vi "CleanupCallback.vi"(8 "error in (no error)":errorcluster, 11 "References":T1) -> (0 "error out":errorcluster)   [LabVIEW 2011]
uses:
  FunctionPointerProxy/LabVIEW/t_CallbackReferences.ctl
  C:/Users/Behavior Room/Desktop/Kinect Mouse/DepthSense/FunctionPointerProxy/FunctionPointerProxy/bin/Release/FunctionPointerProxy.dll
  FunctionPointerProxy/FunctionPointerProxy/bin/Release/FunctionPointerProxy.dll
panel:
  # "//Copyright (c) 2006 Bruno van Dooren\n//Permission is hereby granted, free of charge, to any person obtaining a copy\n//of this software and associated documentation files (the \"Software\"), to deal\n//in the Software without restriction, including without limitation the rights\n//to use, copy, modify, merge, publish, distribute, sublicense, and/or sell\n//copies of the Software, and to permit persons to whom the Software is\n//furnished to do so, subject to the following conditions:\n//The above copyright notice and this permission notice shall be included in all\n//copies or substantial portions of the Software.\n//THE SOFTWARE IS PROVIDED \"AS IS\", WITHOUT WARRANTY OF ANY KIND, EXPRESS OR\n//IMPLIED, INCLUDING BUT NOT LIMITED TO THE WARRANTIES OF MERCHANTABILITY,\n//FITNESS FOR A PARTICULAR PURPOSE AND NONINFRINGEMENT. IN NO EVENT SHALL THE\n//AUTHORS OR COPYRIGHT HOLDERS BE LIABLE FOR ANY CLAIM, DAMAGES OR OTHER\n//LIABILITY, WHETHER IN AN ACTION OF CONTRACT, TORT OR OTHERWISE, ARISING FROM,\n//OUT OF OR IN CONNECTION WITH THE SOFTWARE OR THE USE OR OTHER DEALINGS IN THE\n//SOFTWARE."
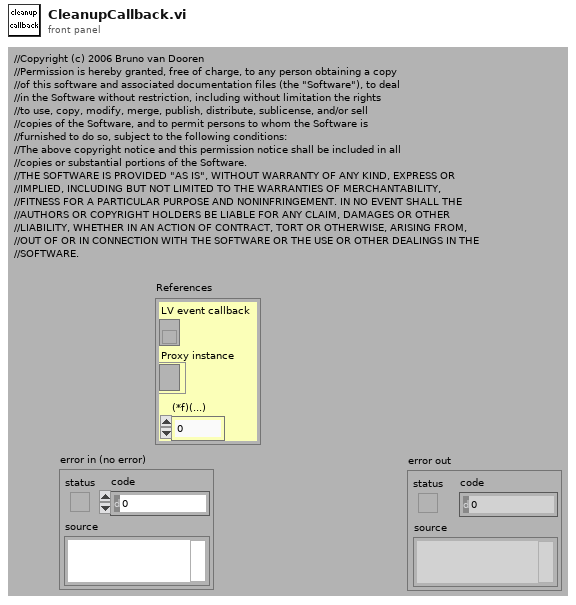
[diagram p1: front panel]
types:
  T1 = typedef "t_CallbackReferences.ctl" = cluster{"LV event callback ":refnum<k27>, "Proxy instance":refnum<k24>, "(*f)(...)":i32}
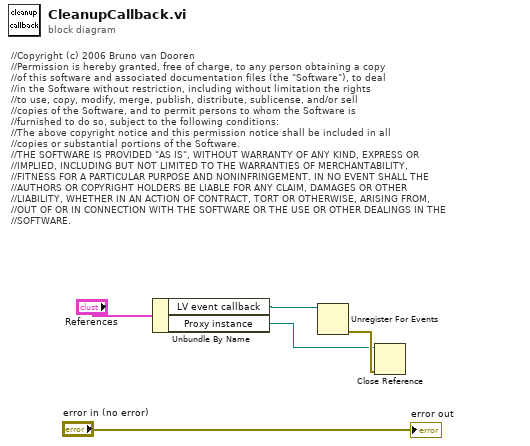
[diagram p0: block diagram]
diagram:
  # "//Copyright (c) 2006 Bruno van Dooren\n//Permission is hereby granted, free of charge, to any person obtaining a copy\n//of this software and associated documentation files (the \"Software\"), to deal\n//in the Software without restriction, including without limitation the rights\n//to use, copy, modify, merge, publish, distribute, sublicense, and/or sell\n//copies of the Software, and to permit persons to whom the Software is\n//furnished to do so, subject to the following conditions:\n//The above copyright notice and this permission notice shall be included in all\n//copies or substantial portions of the Software.\n//THE SOFTWARE IS PROVIDED \"AS IS\", WITHOUT WARRANTY OF ANY KIND, EXPRESS OR\n//IMPLIED, INCLUDING BUT NOT LIMITED TO THE WARRANTIES OF MERCHANTABILITY,\n//FITNESS FOR A PARTICULAR PURPOSE AND NONINFRINGEMENT. IN NO EVENT SHALL THE\n//AUTHORS OR COPYRIGHT HOLDERS BE LIABLE FOR ANY CLAIM, DAMAGES OR OTHER\n//LIABILITY, WHETHER IN AN ACTION OF CONTRACT, TORT OR OTHERWISE, ARISING FROM,\n//OUT OF OR IN CONNECTION WITH THE SOFTWARE OR THE USE OR OTHER DEALINGS IN THE\n//SOFTWARE."
  n1 = Unbundle By Name("References") -> ("LV event callback"=w5:refnum<k27>, "Proxy instance"=w2:refnum<k24>)
  n2 = Unregister For Events(event registration refnum=w5) -> (error out=w3:errorcluster)  [unwired: 1 in]
  n3 = Close Reference(reference=w2, error in (no error)=w3) -> ()  [unwired: 1 out]
  "error out" <- "error in (no error)"
